vi "SetRobotProfile.vi"   [LabVIEW 2023]
doc: "Reads the robot profile from the configuration file on the roboRIO and sets any robot specific parameters."
uses:
  <vilib>/Utility/error.llb/Trim Whitespace One-Sided.vi
  GlobalShooter.vi
  GlobalElevator.vi
  GlobalDrivebase.vi
  GlobalMiscellaneous.vi
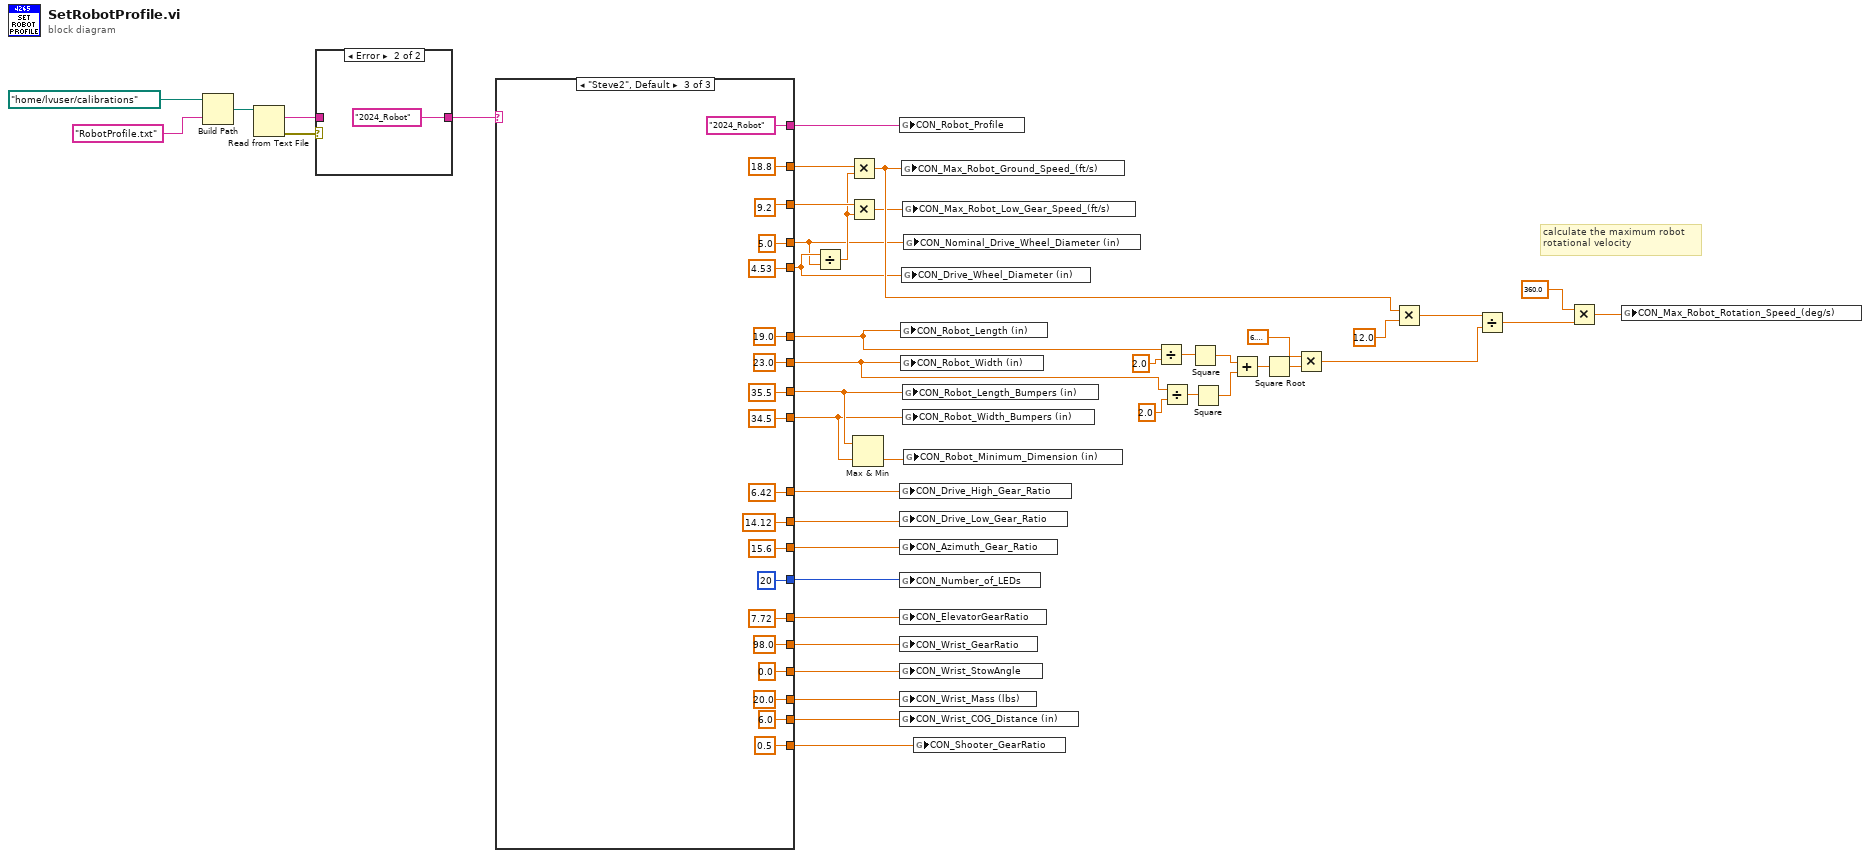
[diagram p0: block diagram]
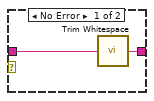
[diagram p2: hidden frame]
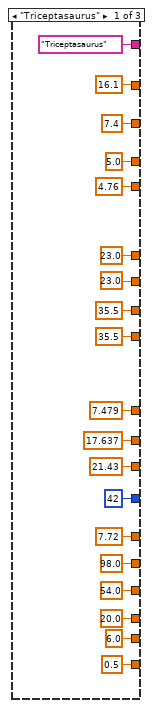
[diagram p3: hidden frame]
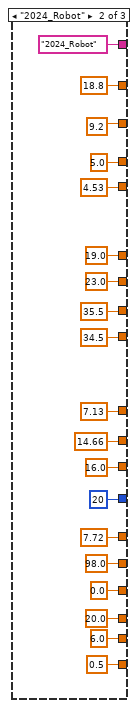
[diagram p4: hidden frame]
diagram:
  # "calculate the maximum robot\nrotational velocity"
  n1 = Build Path(base path=path "/home/lvuser/calibrations" ("path"), name or relative path="RobotProfile.txt") -> (appended path=w43:path)
  n2 = Read from Text File(file (use dialog)=w43) -> (text=w41:string, error out=w42:errorcluster)  [unwired: 3 in, 2 out]
  n3 = case shown="Error" w42 {
    tunnel: w41 -> [w45 _]
    tunnel: [w46 "2024_Robot"] -> w39
    frame No Error {
      n4 = call <vilib>:"Trim Whitespace.vi"("string"=w45) -> ("trimmed string"=w46:string)  [unwired: 1 in]
    }
    frame Error {
    }
  }
  n5 = case shown="\"Steve2\", Default" w39 {
    tunnel: ["Triceptasaurus" "2024_Robot" "2024_Robot"] -> w14
    tunnel: [23.0 ("Robot_Length (in)") 23.0 ("Robot_Length (in)") 23.0 ("Robot_Length (in)")] -> w23
    tunnel: [23.0 ("Robot_Length (in)") 19.0 ("Robot_Length (in)") 19.0 ("Robot_Length (in)")] -> w24
    tunnel: [16.1 ("Max_Robot_Ground_Speed_(ft/s)") 18.8 ("Max_Robot_Ground_Speed_(ft/s)") 18.8 ("Max_Robot_Ground_Speed_(ft/s)")] -> w13
    tunnel: [35.5 ("Robot_Length (in)") 35.5 ("Robot_Length (in)") 35.5 ("Robot_Length (in)")] -> w22
    tunnel: [35.5 ("Robot_Length (in)") 34.5 ("Robot_Length (in)") 34.5 ("Robot_Length (in)")] -> w21
    tunnel: [5.0 ("Robot_Length (in)") 5.0 ("Robot_Length (in)") 5.0 ("Robot_Length (in)")] -> w7
    tunnel: [7.479 ("Robot_Length (in)") 7.13 ("Robot_Length (in)") 6.42 ("Robot_Length (in)")] -> w19
    tunnel: [17.637 ("Robot_Length (in)") 14.66 ("Robot_Length (in)") 14.12 ("Robot_Length (in)")] -> w18
    tunnel: [21.43 ("Robot_Length (in)") 16.0 ("Robot_Length (in)") 15.6 ("Robot_Length (in)")] -> w17
    tunnel: [u16 42 u16 20 u16 20] -> w15
    tunnel: [7.4 ("Max_Robot_Ground_Speed_(ft/s)") 9.2 ("Max_Robot_Ground_Speed_(ft/s)") 9.2 ("Max_Robot_Ground_Speed_(ft/s)")] -> w11
    tunnel: [4.76 ("Robot_Length (in)") 4.53 ("Robot_Length (in)") 4.53 ("Robot_Length (in)")] -> w8
    tunnel: [7.72 7.72 ("Robot_Length (in)") 7.72 ("Robot_Length (in)")] -> w6
    tunnel: [98.0 ("Robot_Length (in)") 98.0 ("Robot_Length (in)") 98.0 ("Robot_Length (in)")] -> w5
    tunnel: [54.0 ("Robot_Length (in)") 0.0 ("Robot_Length (in)") 0.0 ("Robot_Length (in)")] -> w4
    tunnel: [20.0 ("Robot_Length (in)") 20.0 ("Robot_Length (in)") 20.0 ("Robot_Length (in)")] -> w3
    tunnel: [6.0 ("Robot_Length (in)") 6.0 ("Robot_Length (in)") 6.0 ("Robot_Length (in)")] -> w2
    tunnel: [0.5 ("Robot_Length (in)") 0.5 ("Robot_Length (in)") 0.5 ("Robot_Length (in)")] -> w1
    frame "Triceptasaurus" {
    }
    frame "2024_Robot" {
    }
    frame "Steve2", Default {
    }
  }
  n6 = Divide(x=w8, y=w7) -> (x/y=w9:dbl)
  n7 = Multiply(x=w13, y=w9) -> (x*y=w12:dbl)
  n8 = Multiply(x=w11, y=w9) -> (x*y=w10:dbl)
  n9 = Max & Min(x=w22, y=w21) -> (min(x,y)=w20:dbl)  [unwired: 1 out]
  n10 = global write "GlobalMiscellaneous.vi" "CON_Robot_Profile"(w14) -> ()
  n11 = global write "GlobalDrivebase.vi" "CON_Drive_High_Gear_Ratio"(w19) -> ()
  n12 = global write "GlobalDrivebase.vi" "CON_Drive_Low_Gear_Ratio"(w18) -> ()
  n13 = global write "GlobalDrivebase.vi" "CON_Azimuth_Gear_Ratio"(w17) -> ()
  n14 = global write "GlobalMiscellaneous.vi" "CON_Number_of_LEDs"(w15) -> ()
  n15 = global write "GlobalElevator.vi" "CON_ElevatorGearRatio"(w6) -> ()
  n16 = global write "GlobalShooter.vi" "CON_Wrist_GearRatio"(w5) -> ()
  n17 = global write "GlobalShooter.vi" "CON_Wrist_StowAngle"(w4) -> ()
  n18 = global write "GlobalShooter.vi" "CON_Wrist_Mass (lbs)"(w3) -> ()
  n19 = global write "GlobalShooter.vi" "CON_Wrist_COG_Distance (in)"(w2) -> ()
  n20 = global write "GlobalDrivebase.vi" "CON_Robot_Length (in)"(w24) -> ()
  n21 = global write "GlobalDrivebase.vi" "CON_Robot_Width (in)"(w23) -> ()
  n22 = global write "GlobalDrivebase.vi" "CON_Max_Robot_Ground_Speed_(ft/s)"(w12) -> ()
  n23 = global write "GlobalDrivebase.vi" "CON_Drive_Wheel_Diameter (in)"(w8) -> ()
  n24 = global write "GlobalDrivebase.vi" "CON_Max_Robot_Low_Gear_Speed_(ft/s)"(w10) -> ()
  n25 = global write "GlobalDrivebase.vi" "CON_Robot_Length_Bumpers (in)"(w22) -> ()
  n26 = global write "GlobalDrivebase.vi" "CON_Robot_Width_Bumpers (in)"(w21) -> ()
  n27 = global write "GlobalDrivebase.vi" "CON_Nominal_Drive_Wheel_Diameter (in)"(w7) -> ()
  n28 = global write "GlobalDrivebase.vi" "CON_Robot_Minimum_Dimension (in)"(w20) -> ()
  n29 = global write "GlobalShooter.vi" "CON_Shooter_GearRatio"(w1) -> ()
  n30 = Divide(x=w24, y=2.0) -> (x/y=w30:dbl)
  n31 = Divide(x=w23, y=2.0) -> (x/y=w29:dbl)
  n32 = Square(x=w30) -> (x^2=w28:dbl)
  n33 = Square(x=w29) -> (x^2=w27:dbl)
  n34 = Add(x=w28, y=w27) -> (x+y=w26:dbl)
  n35 = Square Root(x=w26) -> (sqrt(x)=w25:dbl)
  n36 = Multiply(x=6.283185307179586, y=w25) -> (x*y=w35:dbl)
  n37 = Multiply(x=w12, y=12.0) -> (x*y=w37:dbl)
  n38 = Divide(x=w37, y=w35) -> (x/y=w34:dbl)
  n39 = Multiply(x=360.0, y=w34) -> (x*y=w16:dbl)
  n40 = global write "GlobalDrivebase.vi" "CON_Max_Robot_Rotation_Speed_(deg/s)"(w16) -> ()
